vi "binToDec.vi"(1 "Array 2":i32[](array[numeric])) -> (0 "output":i32)   [LabVIEW 2020]
panel:
  out "Array":i32[](array[numeric])
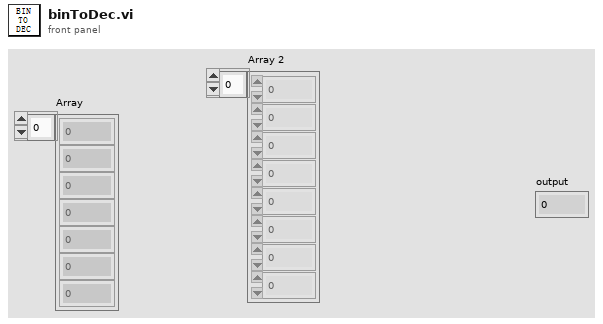
[diagram p1: front panel]
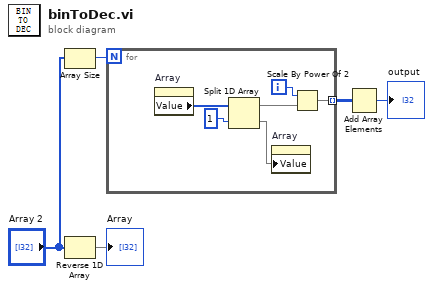
[diagram p0: block diagram]
diagram:
  n1 = Array Size(array="Array 2") -> (size(s)=w3:i32)
  n2 = Reverse 1D Array(array="Array 2") -> (reversed array=→"Array":i32[])
  n3 = for {
    N: w3 -> [_]
    tunnel: [w10] -> w5 mode=indexing
    i -> [w11]
    n4 = property on="Array" class="Arr (strict)"() -> ("Value"=w8:i32[])  [unwired: 2 in, 2 out]
    n5 = Split 1D Array(array=w8, index=1) -> (first subarray=w7:i32[], second subarray=w6:i32[])
    n6 = property on="Array" class="Arr (strict)"("Value"=w6) -> ()  [unwired: 2 in, 2 out]
    n7 = Scale By Power Of 2(n=w11, x=w7) -> (x*2^n=w10:i32[])
  }
  n8 = Add Array Elements(numeric array=w5) -> (sum=→"output":i32)
